vi "显示即时帮助.vi"(8 "error in (no error)":errorcluster caption="错误输入（无错误）", 11 "程序 输入":refnum<class "程序.lvclass">) -> (0 "error out":errorcluster caption="错误输出", 3 "程序 输出":refnum<class "程序.lvclass">)   [LabVIEW 2018, in "程序.lvclass"]
uses:
  <vilib>/Utility/miscctls.llb/LVPositionTypeDef.ctl
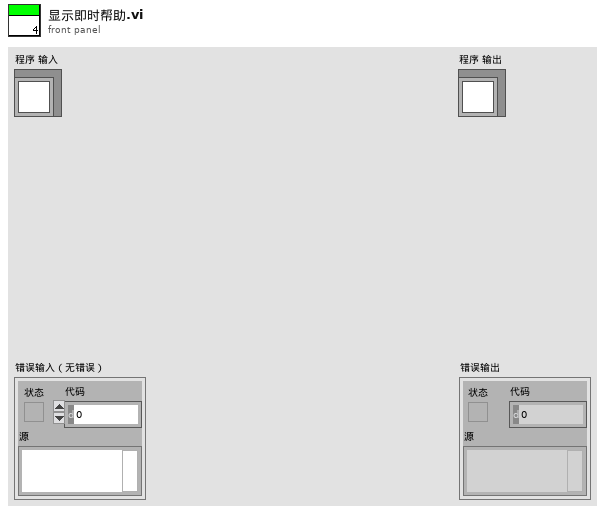
[diagram p1: front panel]
types:
  T1 = typedef "LVPositionTypeDef.ctl" = cluster{"Left":i32, "Top":i32}
  T2 = typedef "LVRectTypeDef.ctl" = cluster{"Left":i16, "Top":i16, "Right":i16, "Bottom":i16}
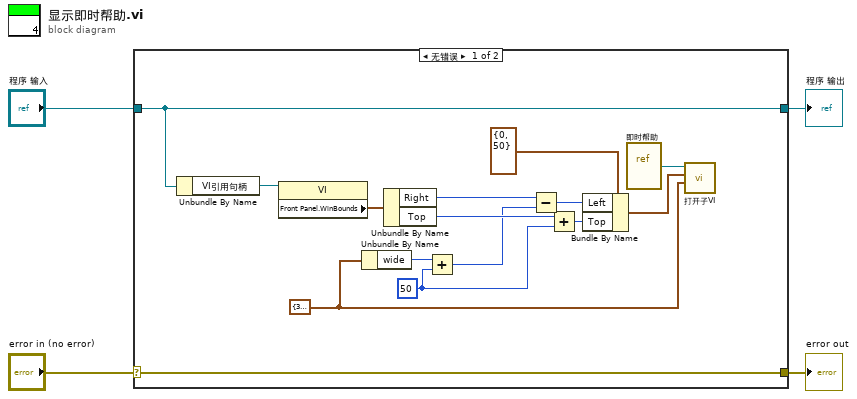
[diagram p0: block diagram]
diagram:
  n1 = case shown="无错误" "error in (no error)" {
    selector: "error in (no error)" -> [w19 w21]
    tunnel: [w19 w21] -> w3
    tunnel: [w17 w20] -> w1
    tunnel: "程序 输入" -> [w17 w20]
    frame No Error {
      w6 = 50 ("y")
      w13 = cluster{"wide":i32, "Top":i32} {"wide"=360, "Top"=318} ("窗口大小")
      n2 = Unbundle By Name(w17) -> ("VI引用句柄"=w16:refnum<vi>)
      n3 = property class="VI"(reference=w16) -> ("Front Panel.WinBounds"=w11:T2)  [unwired: 1 in, 2 out]
      n4 = Unbundle By Name(w13) -> ("wide"=w8:i32)
      n5 = Unbundle By Name(w11) -> ("Right"=w10:i16, "Top"=w9:i16)
      n6 = Add(x=w8, y=w6) -> (x+y=w7:i32)
      n7 = Subtract(x=w10, y=w7) -> (x-y=w12:i32)
      n8 = Add(x=w9, y=w6) -> (x+y=w5:i32)
      n9 = Bundle By Name(cluster=T1 {"Left"=0, "Top"=50} ("窗口位置"), "Left"=w12, "Top"=w5) -> (w14:T1)
      n10 = vi-ref "即时帮助.vi"() -> (w18:refnum<vi>)
      n11 = call "打开子VI.vi"("窗口大小"=w13, "窗口位置"=w14, "引用"=w18) -> ()  [unwired: 7 in, 2 out]
    }
    frame Error {
    }
  }
  "error out" <- w3
  "程序 输出" <- w1
